vi "Output Protection Status.vi"(8 "error in (no error)":errorcluster, 10 "Channel (0: Channel 1)":i32(ring) items=["Channel 1", "Channel 2"], 11 "VISA resource name":refnum<visa-resource-name>) -> (0 "error out":errorcluster, 1 "OCP Tripped?":bool, 2 "OVP Tripped?":bool, 3 "VISA resource name out":refnum<visa-resource-name>)   [LabVIEW 2020, in "Agilent B2900 Series.lvlib"]
doc: "Returns over voltage protection (OVP) and over current protection (OCP) status for a desired channel."
uses:
  Agilent B2900 Series.lvlib
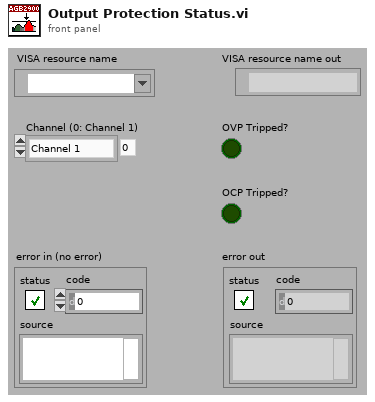
[diagram p1: front panel]
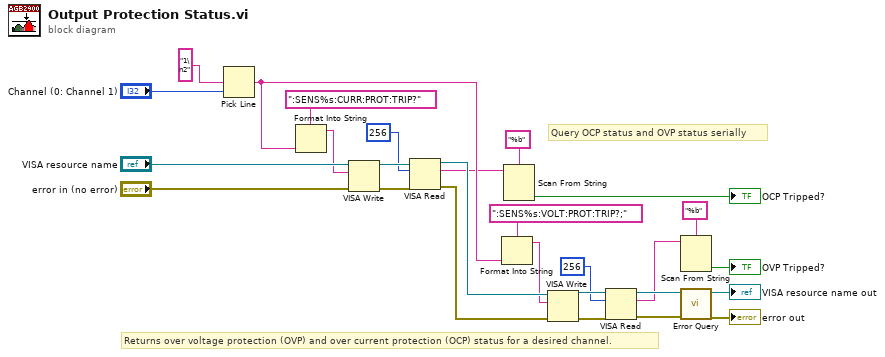
[diagram p0: block diagram]
diagram:
  # "Returns over voltage protection (OVP) and over current protection (OCP) status for a desired channel."
  # "Query OCP status and OVP status serially"
  n1 = Pick Line(multi-line string="1\n2" ("string (\"\")"), line index="Channel (0: Channel 1)") -> (output string=w11:string)  [unwired: 1 in]
  n2 = Format Into String(format string=":SENS%s:CURR:PROT:TRIP?", w11) -> (resulting string=w10:string)  [unwired: 2 in, 1 out]
  n3 = VISA Write(VISA resource name="VISA resource name", write buffer=w10, error in (no error)="error in (no error)") -> (VISA resource name out=w16:refnum<visa-resource-name>, error out=w15:errorcluster)  [unwired: 1 out]
  n4 = VISA Read(VISA resource name=w16, byte count=u32 256, error in (no error)=w15) -> (VISA resource name out=w14:refnum<visa-resource-name>, read buffer=w7:string, error out=w13:errorcluster)  [unwired: 1 out]
  n5 = Format Into String(format string=":SENS%s:VOLT:PROT:TRIP?;", w11) -> (resulting string=w9:string)  [unwired: 2 in, 1 out]
  n6 = Scan From String(format string="%b", input string=w7) -> (output 1=→"OCP Tripped?":bool)  [unwired: 3 in, 3 out]
  n7 = VISA Write(VISA resource name=w14, write buffer=w9, error in (no error)=w13) -> (VISA resource name out=w17:refnum<visa-resource-name>, error out=w20:errorcluster)  [unwired: 1 out]
  n8 = VISA Read(VISA resource name=w17, byte count=u32 256, error in (no error)=w20) -> (VISA resource name out=w18:refnum<visa-resource-name>, read buffer=w3:string, error out=w19:errorcluster)  [unwired: 1 out]
  n9 = Scan From String(format string="%b", input string=w3) -> (output 1=→"OVP Tripped?":bool)  [unwired: 3 in, 3 out]
  n10 = call "Error Query.vi"("error in (no error)"=w19, "VISA resource name"=w18) -> ("error out"=→"error out":errorcluster, "VISA resource name out"=→"VISA resource name out":refnum<visa-resource-name>)  [unwired: 6 in, 2 out]
